vi "Liquid Unit Detect.vi"(7 "Unit ID (A)":string="A", 8 "error in":errorcluster, 11 "VISA Session In":refnum<visa-resource-name>="Alicat") -> (0 "error out":errorcluster, 2 "Liquid Device":bool, 3 "VISA Session Out":refnum<visa-resource-name>)   [LabVIEW 2015]
doc: "Determines if the device connected is a liquid unit."
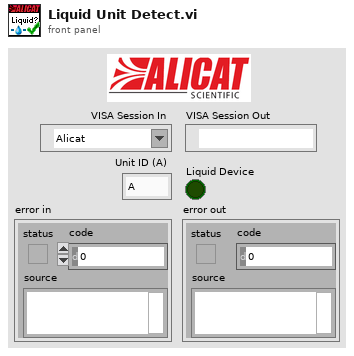
[diagram p1: front panel]
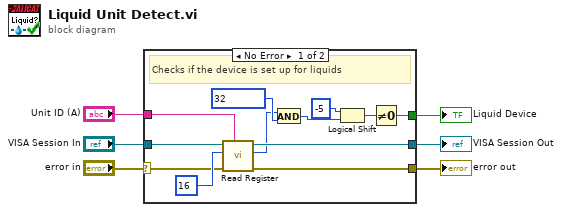
[diagram p0: block diagram]
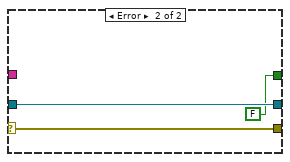
[diagram p2: hidden frame]
diagram:
  n1 = case shown="No Error" "error in" {
    selector: "error in" -> [w7 w19]
    tunnel: "VISA Session In" -> [w14 w21]
    tunnel: "Unit ID (A)" -> [w13 _]
    tunnel: [w12 w19] -> w4
    tunnel: [w11 w21] -> w3
    tunnel: [w8 FALSE] -> w2
    frame No Error {
      # "Checks if the device is set up for liquids"
      n2 = call "Read Register.vi"("Unit ID (A)"=w13, "error in"=w7, "Register address"=u16 16 ("register"), "VISA Session In"=w14) -> ("error out"=w12:errorcluster, "Register Value (I32)"=w10:i32, "VISA Session Out"=w11:refnum<visa-resource-name>)  [unwired: 5 in]
      n3 = And(x=w10, y=32) -> (x .and. y?=w18:i32)
      n4 = Logical Shift(y=i16 -5, x=w18) -> (x << y=w9:i32)
      n5 = Not Equal To 0?(x=w9) -> (x != 0?=w8:bool)
    }
    frame Error {
    }
  }
  "error out" <- w4
  "VISA Session Out" <- w3
  "Liquid Device" <- w2
